vi "Intake Loop.vi"   [LabVIEW 2015]
uses:
  Robot Global Data.vi
types:
  T1 = typedef "Dashboard Control Data.ctl" = cluster{"Encoder Control":T2, "Steer PID output":cluster{"output high":dbl, "output low":dbl}, " Steer PID gains":cluster{"proportional gain (Kc)":dbl, "integral time (Ti, min)":dbl, "derivative time (Td, min)":dbl}, "Drivetrain Settings":T3, "Vision Packet":T4, "Dashboard Drivetrain Command":T5, "Info/Command Cluster":T7, "Ball Vision Packet":T8, "Intake Presets":T10, "Intake Encoder Control":T12, "Goal Output Range":cluster{"output high":dbl, "output low":dbl}, "Enabled Systems":T13, "Auton Presets":T14, "Pressure M":dbl, "Pressure B":dbl, "Vision Timeout":dbl, "Auto-Shift":T15, "Catapult Setpoints":T16, "Climb Presets":T17}
  T2 = typedef "Encoder Control.ctl" = cluster{"Right Tick Constant":dbl, "Left Tick Constant":dbl, "Reset?":bool, "Y Dist":cluster{"PID gains":cluster{"proportional gain (Kc)":dbl, "integral time (Ti, min)":dbl, "derivative time (Td, min)":dbl}}, "Y Stop Thresh":dbl, "Y Stop Speed":dbl}
  T3 = typedef "Drivetrain Settings.ctl" = cluster{"Gyro Tolerance":dbl, "Throttle Ramp (ms)":dbl, "Kv":dbl, "Ka":dbl, "Feed Forward P":dbl, "Feed Forward D":dbl, "Goal Vision PID gains":cluster{"proportional gain (Kc)":dbl, "integral time (Ti, min)":dbl, "derivative time (Td, min)":dbl}, "Goal Detection Window":dbl, "Creep Rate":dbl, "Vision Throttle Threshold":dbl, "Min Turn Output":dbl, "Left Batter Angle":dbl, "Right Batter Angle":dbl}
  T4 = typedef "Goal Vision Packet.ctl" = cluster{"Distance":dbl, "Center X":dbl, "Center Y":dbl, "Found Target?":bool, "Robot Center":dbl, "Angle":dbl}
  T5 = typedef "Dashboard Drivetrain Command.ctl" = cluster{"Drivetrain Vision":T6}
  T6 = typedef "Drivetrain Vision.ctl" = cluster{"Goal Window":dbl, "Ball Window":dbl}
  T7 = typedef "Ball Tracking Command Cluster.ctl" = cluster{"Distance to Ball":dbl, "Desired Angle":dbl, "Command":enum16{"Turn to Ball", "Turn to Angle", "Get Distance"}, "Pixels from Center":dbl}
  T8 = typedef "Ball Vision Packet.ctl" = cluster{"Ball Detected?":bool, "Distance to Ball":dbl, "Desired Angle":dbl, "Pixels from Center":dbl, "Tracking mode":T9}
  T9 = typedef "Tracking Mode.ctl" = enum16{"Turn to Ball", "Turn to Angle"}
  T10 = typedef "Intake Presets.ctl" = cluster{"Intake Speed":dbl, "Outake Speed":dbl, "Angle Speed":dbl, "Angle Tolerance":dbl, "Encoder Scale":dbl, "Load Height":dbl, "Output Range":T11, "MaxCurrent":dbl, "Idle Height":dbl, "Max Height":dbl, "Reset Encoders?":bool, "PID gains":cluster{"proportional gain (Kc)":dbl, "integral time (Ti, min)":dbl, "derivative time (Td, min)":dbl}, "Drop Low Height ":dbl, "Rotation Power Max/Min":dbl, "Reset Delay":dbl, "Current Trip Delay":dbl}
  T11 = typedef "Drivetrain Output Range.ctl" = cluster{"output high":dbl, "output low":dbl}
  T12 = typedef "IntakeEcoderControl.ctl" = cluster{"Arm Tick Constant":dbl, "Reset?":bool, "Y Dist":cluster{"PID gains":cluster{"proportional gain (Kc)":dbl, "integral time (Ti, min)":dbl, "derivative time (Td, min)":dbl}}, "Y Stop Thresh":dbl, "Y Stop Speed":dbl}
  T13 = typedef "Enabled Systems.ctl" = cluster{"Shoot":bool, "Intake":bool, "DT":bool, "Gyro":bool, "100ms":bool, "US":bool}
  T14 = typedef "Autonomous Presets.ctl" = cluster{"Pitch Limit":dbl, "Roll Limit":dbl, "Start Position":dbl, "Cross Position":dbl}
  T15 = typedef "Auto Shift Cluster.ctl" = cluster{"Delay":dbl, "Speed Thresh":dbl, "Upshift Accel":dbl, "Upshift Throttle":dbl, "Upshift Throttle Accel":dbl, "Downshift Throttle":dbl, "Downshift Throttle Accel":dbl, "Pressure Threshold":dbl}
  T16 = typedef "Catapult Presets.ctl" = cluster{"Intake Danger Height":dbl, "Ball Security Delay ":dbl, "High PSI Minimum":dbl, "Shot Finish Delay":dbl, "Low PSI Minimum":dbl, "Idle Ball Security Wait ":dbl}
  T17 = typedef "Climb Presets.ctl" = cluster{"Winch Speed":dbl, "Wait until Fire":dbl, "Wait until Winch":dbl, "Wait until Stop":dbl}
  T18 = typedef "Intake Commands Cluster.ctl" = cluster{"Intake Commands":T19, "Intake Mode":T20}
  T19 = typedef "Intake Commands.ctl" = enum16{"Zero", "Unload", "Load", "Drop low", "Idle"}
  T20 = typedef "Intake Mode.ctl" = enum16{"Manual", "Safe", "Auto"}
  T21 = typedef "WPI_MotorControlDeviceRef.ctl" = cluster{"DeviceStatus":errorcluster, "Type":T22, "PWM":cluster{"PWM Channel":T23, "DeadBand":T24}, "CAN":cluster{"Device Number":u8, "Control Mode":T25, "Semaphore":T26, "Max Vout":dbl, "TalonSRX Control Mode":T27}, "Invert":bool}
  T22 = typedef "WPI_MotorControlType.ctl" = enum16{"PWM", "CAN", "CANTalonSRX"}
  T23 = typedef "FPGA_DIOPWMChannel.ctl" = enum8{"PWM 0", "PWM 1", "PWM 2", "PWM 3", "PWM 4", "PWM 5", "PWM 6", "PWM 7", "PWM 8", "PWM 9", "PWM MXP 0", "PWM MXP 1", "PWM MXP 2", "PWM MXP 3", "PWM MXP 4", "PWM MXP 5", "PWM MXP 6", "PWM MXP 7", "PWM MXP 8", "PWM MXP 9", "Invalid"}
  T24 = typedef "WPI_PWMDeadband.ctl" = cluster{"Name":string, "maxPositivePwm":i32, "minPositivePwm":i32, "centerPwm":i32, "maxNegativePwm":i32, "minNegativePwm":i32, "angularRange":u16}
  T25 = typedef "WPI_CANJaguar_ControlMode.ctl" = enum8{"Percent VBus", "Current", "Speed", "Position", "Voltage"}
  T26 = typedef "Semaphore RefNum" = refnum<k1>
  T27 = typedef "WPI_CANTalonSRX_APIControlMode.ctl" = enum8{"Percent VBus", "Speed", "Position", "Slave", "Unchanged / Invalid", "Voltage Compensation", "Current", "Motion Profile"}
  T28 = typedef "WPI_CANTalonSRX_GlobalStatus.ctl" = cluster{"Applied Throttle":dbl, "Module Enabled":bool, "CAN Error":errorcluster, "Closed Loop Error":dbl, "Forward Limit Switch Closed":bool, "Reverse Limit Switch Closed":bool, "Sensor Position":dbl, "Sensor Velocity":dbl, "Current":dbl, "Sticky Fault - Over Temp":bool, "Sticky Fault - Under Voltage":bool, "Sticky Fault - Forward Limit":bool, "Sticky Fault - Reverse Limit":bool, "Sticky Fault - Forward Soft Limit":bool, "Sticky Fault - Reverse Soft Limit":bool, "Brake is Enabled":bool, "Encoder Position":dbl, "Encoder Velocity":dbl, "Encoder Index Count":dbl, "Encoder A Pin State":bool, "Encoder B Pin State":bool, "Encoder Index Pin State":bool, "Analog In":dbl, "Analog In Velocity":dbl, "Temperature (C)":dbl, "Battery Voltage":dbl, "Control 5 Is Supported":bool, "Current Profile Slot Select":dbl, "Pos Div 8":bool, "Vel Div 4":bool, "Pulse Width Position":i32, "Pulse Width Velocity":i32, "Pulse Width Rise To Rise (us)":i32, "Pulse Width Rise To Fall (us)":i32, "Mot Prof Active Is Under Run":bool, "Mot Prof Active Has Under Run":bool, "Mot Prof Active Is Last":bool, "Mot Prof Active Velocity Only":bool, "Mot Prof Active Is Valid":bool, "Mot Prof Buffer Is Full":bool, "Mot Prof Active Profile Slot Select":i32, "Mot Prof NextID":i32, "Mot Prof Count":i32, "Mot Prof Active Velocity":dbl, "Mot Prof Active Position":dbl, "Mot Prof Output Enable":i32}
  T29 = typedef "Intake Status Cluster.ctl" = cluster{"Roller Power":dbl, "Angle Power":dbl, "Intake Mode":T20, "Rollers Active?":bool, "Current Height":dbl, "Target Height":dbl, "Encoder Raw Position":dbl, "Forward Tripped?":bool, "Backward Tripped?":bool, "Override IR?":bool, "Intake State":T19}
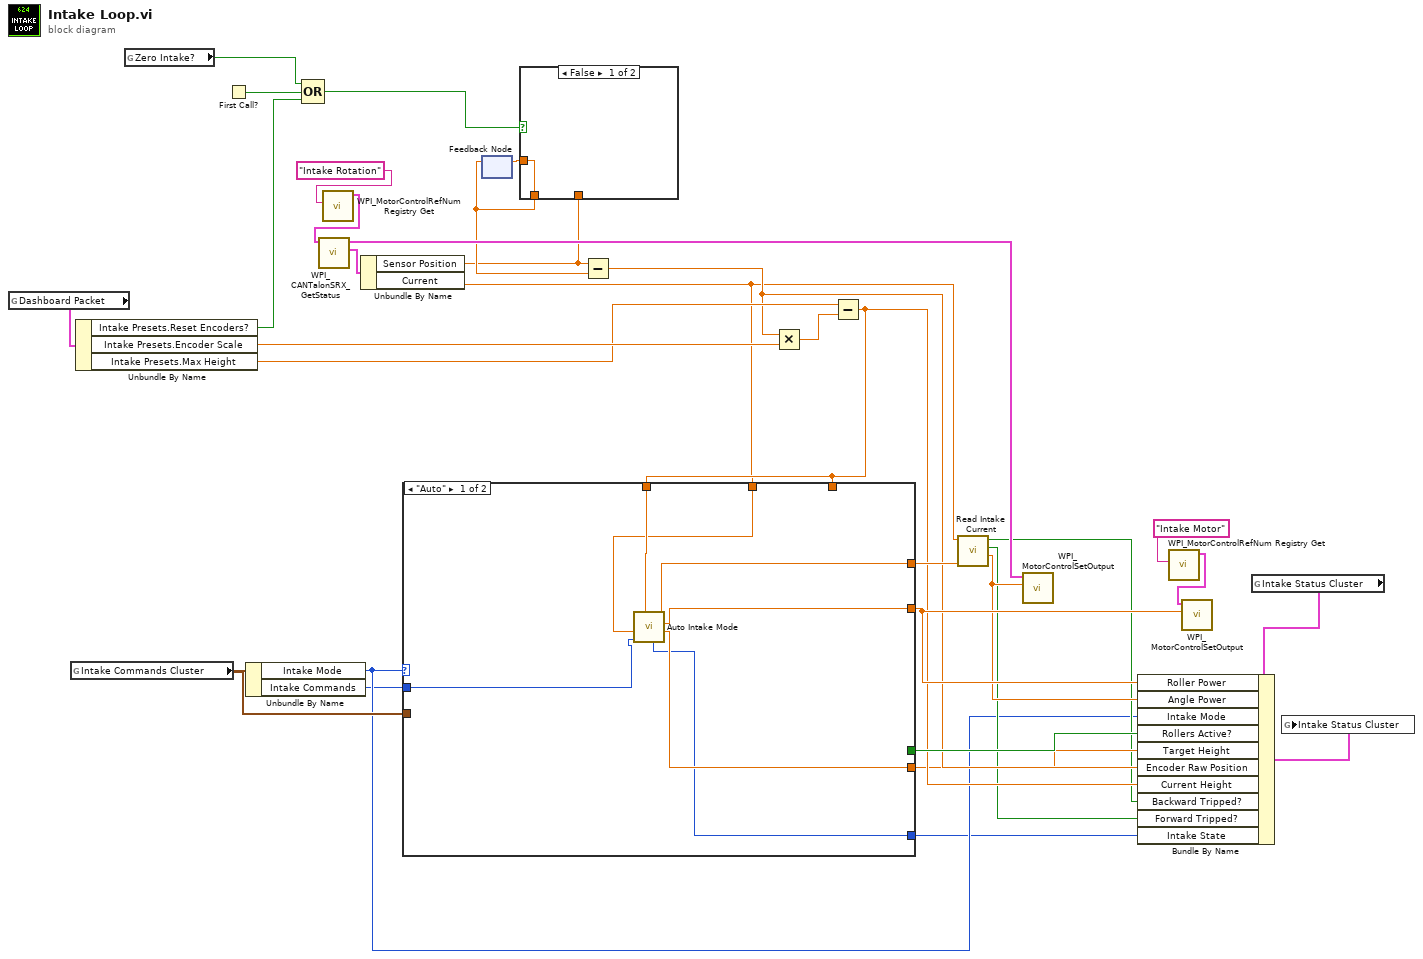
[diagram p0: block diagram]
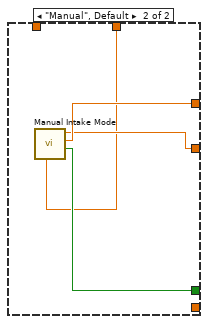
[diagram p3: hidden frame]
diagram:
  n1 = global read "Robot Global Data.vi" "Dashboard Packet"() -> (w20:T1)
  n2 = global read "Robot Global Data.vi" "Intake Commands Cluster"() -> (w33:T18)
  n3 = Unbundle By Name(w20) -> ("Intake Presets.Reset Encoders?"=w11:bool, "Intake Presets.Encoder Scale"=w22:dbl, "Intake Presets.Max Height"=w21:dbl)
  n4 = global read "Robot Global Data.vi" "Zero Intake?"() -> (w8:bool)
  n5 = First Call?() -> (First Call?: T/F=w10:bool)
  n6 = Unbundle By Name(w33) -> ("Intake Mode"=w3:T20, "Intake Commands"=w2:T19)
  n7 = Compound Arithmetic op=OR(w8, w10, w11) -> (w9:bool)
  n8 = call <vilib>:"WPI_MotorControlRefNum Registry Get.vi"("refnum name"="Intake Rotation") -> ("MotorControlDevRef"=w17:T21)  [unwired: 9 in, 1 out]
  n9 = call <vilib>:"WPI_CANTalonSRX_GetStatus.vi"("CAN Talon SRX Ref"=w17) -> ("Talon SRX Status"=w19:T28, "CAN Talon SRX Ref"=w18:T21)  [unwired: 8 in, 1 out]
  n10 = Unbundle By Name(w19) -> ("Sensor Position"=w14:dbl, "Current"=w6:dbl)
  n11 = feedback #1() -> (w15:dbl)  [unwired: 1 in]
  n12 = case shown="False" w9 {
    tunnel: w14 -> [_ w35]
    tunnel: [w34 w35] -> w16
    tunnel: w15 -> [w34 _]
    frame False {
    }
    frame True {
    }
  }
  n13 = feedback-in #1(w16) -> ()
  n14 = Subtract(x=w14, y=w15) -> (x-y=w13:dbl)
  n15 = Multiply(x=w13, y=w22) -> (x*y=w23:dbl)
  n16 = Subtract(x=w21, y=w23) -> (x-y=w12:dbl)
  n17 = case shown="\"Auto\"" w3 {
    tunnel: w33 -> [_ _]
    tunnel: [w39 w46] -> w26
    tunnel: [w40 w45] -> w30
    tunnel: w12 -> [_ w43]
    tunnel: [_ w44] -> w24
    tunnel: w12 -> [w42 _]
    tunnel: [w41 _] -> w7
    tunnel: w6 -> [w38 _]
    tunnel: w2 -> [w37 _]
    tunnel: [w36 _] -> w1
    frame "Auto" {
      n18 = call "Auto Intake Mode.vi"("Intake Current Angle"=w42, "Intake Commands"=w37, "Current"=w38) -> ("Target Height"=w41:dbl, "Roller Speed"=w40:dbl, "Angle Power"=w39:dbl, "Intake States"=w36:T19)  [unwired: 5 in]
    }
    frame "Manual", Default {
      n19 = call "Manual Intake Mode.vi"("Current Encoder Position"=w43) -> ("Rollers Active?"=w44:bool, "Arm Power"=w46:dbl, "Intake Power"=w45:dbl)  [unwired: 8 in]
    }
  }
  n20 = call "Read Intake Current.vi"("Proposed Power"=w26, "Current"=w6) -> ("Actual Power"=w25:dbl, "Forward Trip"=w4:bool, "Backward Trip"=w5:bool)  [unwired: 7 in]
  n21 = call <vilib>:"WPI_MotorControlSetOutput.vi"("Output"=w25, "MotorControlDevRef"=w18) -> ()  [unwired: 7 in, 3 out]
  n22 = call <vilib>:"WPI_MotorControlRefNum Registry Get.vi"("refnum name"="Intake Motor") -> ("MotorControlDevRef"=w31:T21)  [unwired: 9 in, 1 out]
  n23 = call <vilib>:"WPI_MotorControlSetOutput.vi"("Output"=w30, "MotorControlDevRef"=w31) -> ()  [unwired: 7 in, 3 out]
  n24 = global read "Robot Global Data.vi" "Intake Status Cluster"() -> (w28:T29)
  n25 = Bundle By Name(cluster=w28, "Roller Power"=w30, "Angle Power"=w25, "Intake Mode"=w3, "Rollers Active?"=w24, "Target Height"=w7, "Encoder Raw Position"=w13, "Current Height"=w12, "Backward Tripped?"=w5, "Forward Tripped?"=w4, "Intake State"=w1) -> (w29:T29)
  n26 = global write "Robot Global Data.vi" "Intake Status Cluster"(w29) -> ()
